vi "PUC.vi"() -> ()   [LabVIEW 2024]
uses:
  <instrlib>/OptoMMP/OptoMMP.lvlib
panel:
  out "PUC Error":errorcluster
  in  "IP Address":string
  # "Opto 22 Powerup Clear"
  # "Enter the IP address\nof the Opto 22 device"
  # "Copyright (c) 2025 California Institute of Technology (Caltech).\nU.S. Government sponsorship acknowledged.\n\nLicensed under the Apache License, Version 2.0 (the \"License\");\nyou may not use this file except in compliance with the License.\nYou may obtain a copy of the License at\n\n    http://www.apache.org/licenses/LICENSE-2.0\n\nUnless required by applicable law or agreed to in writing, software\ndistributed under the License is distributed on an \"AS IS\" BASIS,\nWITHOUT WARRANTIES OR CONDITIONS OF ANY KIND, either express or implied.\nSee the License for the specific language governing permissions and\nlimitations under the License."
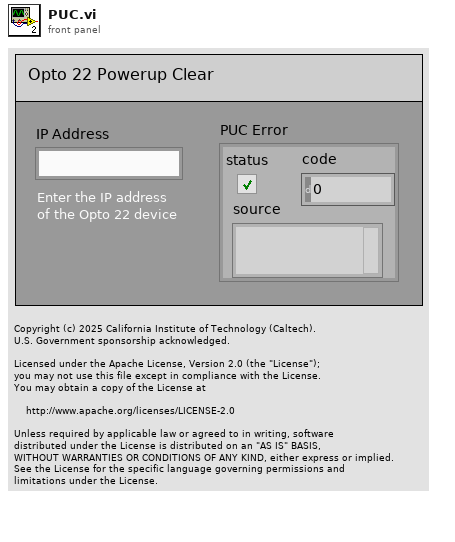
[diagram p1: front panel]
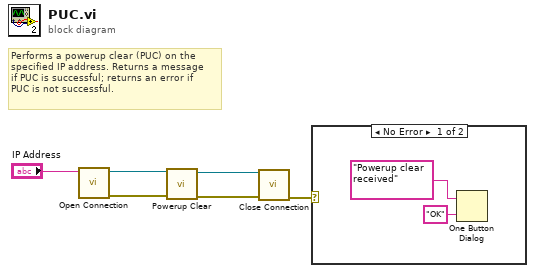
[diagram p0: block diagram]
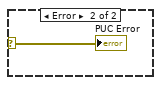
[diagram p2: hidden frame]
diagram:
  # "Performs a powerup clear (PUC) on the \nspecified IP address. Returns a message\nif PUC is successful; returns an error if\nPUC is not successful."
  n1 = call <instrlib>:"Open Connection.vi"("Client IP Address"="IP Address") -> ("error out"=w5:errorcluster, "TCP Network Connection out"=w6:refnum<k5>)  [unwired: 9 in]
  n2 = call <instrlib>:"Powerup Clear.vi"("error in (no error)"=w5, "TCP Network Connection in"=w6) -> ("error out"=w2:errorcluster, "connection ID out"=w3:refnum<k5>)  [unwired: 8 in]
  n3 = call <instrlib>:"Close Connection.vi"("error in (no error)"=w2, "TCP Network Connection in"=w3) -> ("error out"=w1:errorcluster)  [unwired: 8 in, 1 out]
  n4 = case shown="No Error" w1 {
    selector: w1 -> [_ w9]
    frame No Error {
      n5 = One Button Dialog(message="Powerup clear received", button name ("OK")="OK") -> ()  [unwired: 1 out]
    }
    frame Error {
      "PUC Error" <- w9
    }
  }
